vi "solar_cfg String to Variant.vi"(6 "ArrayDelimiters (1D,2D)":string[](array[string]), 8 "error in (no error)":errorcluster, 10 "String":string, 11 "Variant in":variant) -> (0 "error out":errorcluster, 2 "Variant (Binary)":string, 3 "Variant out":variant)   [LabVIEW 2018]
doc: "This converts the ASCII <b>String</b> to <b>Variant out</b> given the <b>Variant in</b> data type."
uses:
  <vilib>/Utility/Data Type/NI_Data Type.lvlib
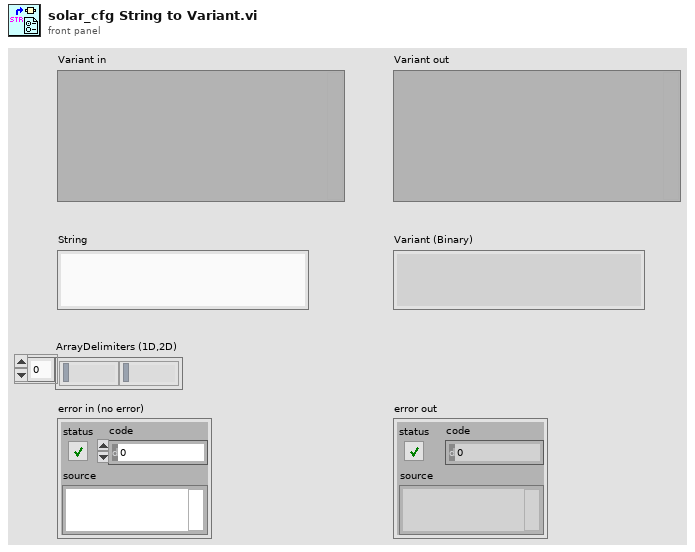
[diagram p1: front panel]
types:
  T1 = typedef "NI_Data Type.lvlib/Data Type.ctl" = enum8{"Invalid Type", "Void", "I8", "I16", "I32", "I64", "U8", "U16", "U32", "U64", "Single Float", "Double Float", "Extended Float", "Single Complex", "Double Complex", "Extended Complex", "Enum U8", "Enum U16", "Enum U32", "Enum U64", "Single Float With Unit", "Double Float With Unit", "Extended Float With Unit", "Single Complex with Unit", "Double Complex with Unit", "Extended Complex with Unit", "Boolean", "String", "Path", "Picture", "Tag", "Array", "Cluster", "Variant", "LV Variant", "Waveform", "Timestamp", "Digital Waveform", "Digital Data", "ExpressData", "Refnum", "External Data", "VI", "Poly VI", "LabVIEW Class Instance", "Fixed Point", "Set Collection", "Map Collection"}
  T2 = typedef "NI_Data Type.lvlib/Refnum Type.ctl" = enum16{"NotARefnum", "UnknownRefnum", "Generic", "Datalog", "ByteStream", "Device", "Occurence", "TCPNetConnection", "Auto", "Menu", "Imaq", "Hardware", "DataSocket", "Visa", "IVI", "UDPNetConnection", "Notifier", "Queue", "Irda", "EventReg", "DotNet", "UserEvent", "Callback", "UNUSED_EMPTY_POSITION", "BlueToothNetConnection", "LVObjApp", "LVObjVI", "LVObjUnknown", "GenericClass", "UserDefinedRefnumTag", "DataValue", "RT FIFO", "TDMS File", "PythonSessionRefnum"}
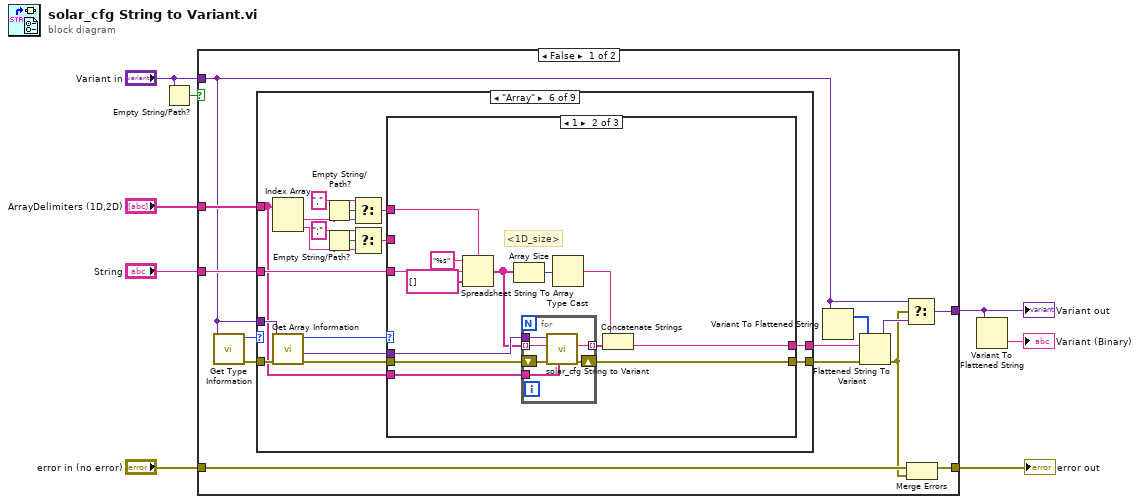
[diagram p0: block diagram]
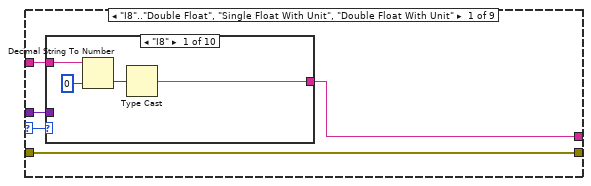
[diagram p2: hidden frame]
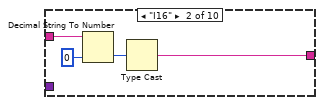
[diagram p3: hidden frame]
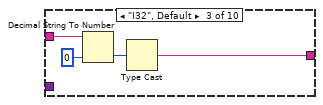
[diagram p4: hidden frame]
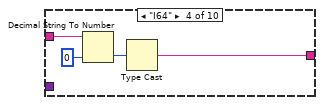
[diagram p5: hidden frame]
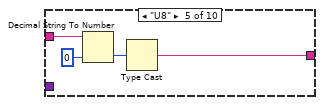
[diagram p6: hidden frame]
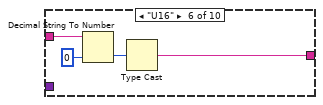
[diagram p7: hidden frame]
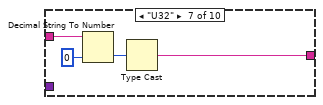
[diagram p8: hidden frame]
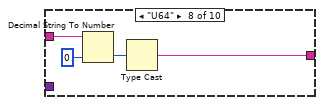
[diagram p9: hidden frame]
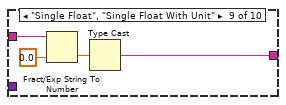
[diagram p10: hidden frame]
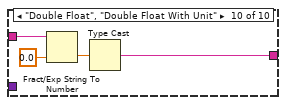
[diagram p11: hidden frame]
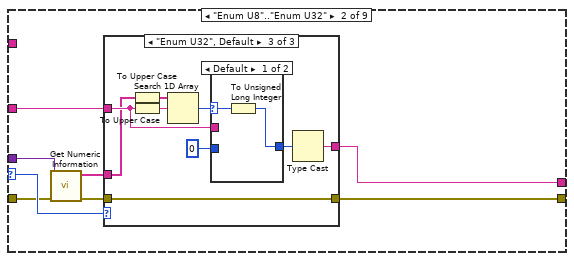
[diagram p12: hidden frame]
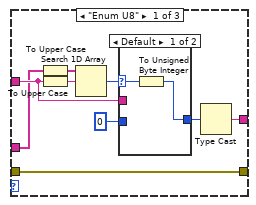
[diagram p13: hidden frame]
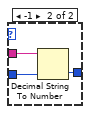
[diagram p14: hidden frame]
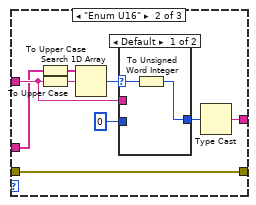
[diagram p15: hidden frame]
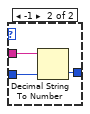
[diagram p16: hidden frame]
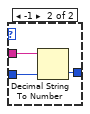
[diagram p17: hidden frame]
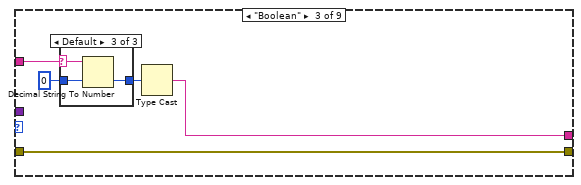
[diagram p18: hidden frame]
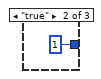
[diagram p20: hidden frame]
diagram:
  n1 = Empty String/Path?(string/path="Variant in") -> (empty?=w1:bool)
  n2 = case shown="False" w1 {
    tunnel: "ArrayDelimiters (1D,2D)" -> [w19 _]
    tunnel: "error in (no error)" -> [w18 w267]
    tunnel: [w17 w267] -> w6
    tunnel: "String" -> [w16 _]
    tunnel: "Variant in" -> [w12 w266]
    tunnel: [w10 w266] -> w3
    frame False {
      n3 = call <vilib>:"Get Type Information.vi"("variant"=w12) -> ("error out"=w20:errorcluster, "type"=w21:T1)  [unwired: 6 in, 3 out]
      n4 = case shown="\"Array\"" w21 {
        selector: w21 -> [w24 w73 _ _ _ _ _ _ _]
        tunnel: w12 -> [w22 w71 _ _ _ w150 _ w229 _]
        tunnel: w20 -> [w26 w72 w118 w128 w135 w153 w223 w230 w258]
        tunnel: [w26 w74 w118 w128 w134 w142 w219 w232 w258] -> w14
        tunnel: [w23 w67 w117 w127 w132 w141 w220 w231 w252] -> w13
        tunnel: w19 -> [_ _ _ _ _ w137 _ _ _]
        tunnel: w16 -> [w25 w68 w119 w129 w133 w139 w222 w226 w253]
        frame "I8".."Double Float", "Single Float With Unit", "Double Float With Unit" {
          n5 = case shown="\"I8\"" w24 {
            tunnel: w25 -> [w28 w32 w36 w40 w44 w48 w52 w56 w61 w65]
            tunnel: [w27 w31 w35 w39 w43 w47 w51 w55 w62 w66] -> w23
            tunnel: w22 -> [_ _ _ _ _ _ _ _ _ _]
            frame "I8" {
              n6 = Decimal String To Number(string=w28, default (0L)=i8 0 ("default (0 I32)")) -> (number=w29:i8)  [unwired: 1 in, 1 out]
              n7 = Type Cast(x=w29) -> (*(type *) &x=w27:string)  [unwired: 1 in]
            }
            frame "I16" {
              n8 = Decimal String To Number(string=w32, default (0L)=i16 0 ("default (0 I32)")) -> (number=w33:i16)  [unwired: 1 in, 1 out]
              n9 = Type Cast(x=w33) -> (*(type *) &x=w31:string)  [unwired: 1 in]
            }
            frame "I32", Default {
              n10 = Decimal String To Number(string=w36, default (0L)=0 ("default (0 I32)")) -> (number=w37:i32)  [unwired: 1 in, 1 out]
              n11 = Type Cast(x=w37) -> (*(type *) &x=w35:string)  [unwired: 1 in]
            }
            frame "I64" {
              n12 = Decimal String To Number(string=w40, default (0L)=i64 0 ("default (0 I32)")) -> (number=w41:i64)  [unwired: 1 in, 1 out]
              n13 = Type Cast(x=w41) -> (*(type *) &x=w39:string)  [unwired: 1 in]
            }
            frame "U8" {
              n14 = Decimal String To Number(string=w44, default (0L)=u8 0 ("default (0 I32)")) -> (number=w45:u8)  [unwired: 1 in, 1 out]
              n15 = Type Cast(x=w45) -> (*(type *) &x=w43:string)  [unwired: 1 in]
            }
            frame "U16" {
              n16 = Decimal String To Number(string=w48, default (0L)=u16 0 ("default (0 I32)")) -> (number=w49:u16)  [unwired: 1 in, 1 out]
              n17 = Type Cast(x=w49) -> (*(type *) &x=w47:string)  [unwired: 1 in]
            }
            frame "U32" {
              n18 = Decimal String To Number(string=w52, default (0L)=u32 0 ("default (0 I32)")) -> (number=w53:u32)  [unwired: 1 in, 1 out]
              n19 = Type Cast(x=w53) -> (*(type *) &x=w51:string)  [unwired: 1 in]
            }
            frame "U64" {
              n20 = Decimal String To Number(string=w56, default (0L)=u64 0 ("default (0 I32)")) -> (number=w57:u64)  [unwired: 1 in, 1 out]
              n21 = Type Cast(x=w57) -> (*(type *) &x=w55:string)  [unwired: 1 in]
            }
            frame "Single Float", "Single Float With Unit" {
              n22 = Fract/Exp String To Number(string=w61, default (0 dbl)=sgl 0.0 ("default (0 I32)")) -> (number=w59:sgl)  [unwired: 2 in, 1 out]
              n23 = Type Cast(x=w59) -> (*(type *) &x=w62:string)  [unwired: 1 in]
            }
            frame "Double Float", "Double Float With Unit" {
              n24 = Fract/Exp String To Number(string=w65, default (0 dbl)=0.0 ("default (0 I32)")) -> (number=w63:dbl)  [unwired: 2 in, 1 out]
              n25 = Type Cast(x=w63) -> (*(type *) &x=w66:string)  [unwired: 1 in]
            }
          }
        }
        frame "Enum U8".."Enum U32" {
          n26 = call <vilib>:"Get Numeric Information.vi"("error in (no error)"=w72, "variant"=w71) -> ("error out"=w70:errorcluster, "enum names"=w69:string[])  [unwired: 6 in, 2 out]
          n27 = case shown="\"Enum U32\", Default" w73 {
            tunnel: w70 -> [w77 w91 w105]
            tunnel: [w77 w91 w105] -> w74
            tunnel: w69 -> [w76 w90 w104]
            tunnel: w68 -> [w78 w92 w106]
            tunnel: [w75 w89 w103] -> w67
            frame "Enum U8" {
              n28 = To Upper Case(1:w76) -> (0:w81:string[])
              n29 = To Upper Case(1:w78) -> (0:w80:string)
              n30 = Search 1D Array(1D array=w81, element=w80) -> (index of element=w82:i32)  [unwired: 1 in]
              n31 = case shown="Default" w82 {
                selector: w82 -> [w85 _]
                tunnel: [w84 w88] -> w83
                tunnel: w78 -> [_ w87]
                tunnel: u8 0 ("default (0 I32)") -> [_ w86]
                frame Default {
                  n32 = To Unsigned Byte Integer(number=w85) -> (unsigned 8bit integer=w84:u8)
                }
                frame -1 {
                  n33 = Decimal String To Number(string=w87, default (0L)=w86) -> (number=w88:u8)  [unwired: 1 in, 1 out]
                }
              }
              n34 = Type Cast(x=w83) -> (*(type *) &x=w75:string)  [unwired: 1 in]
            }
            frame "Enum U16" {
              n35 = To Upper Case(1:w90) -> (0:w95:string[])
              n36 = To Upper Case(1:w92) -> (0:w94:string)
              n37 = Search 1D Array(1D array=w95, element=w94) -> (index of element=w96:i32)  [unwired: 1 in]
              n38 = case shown="Default" w96 {
                selector: w96 -> [w99 _]
                tunnel: [w98 w102] -> w97
                tunnel: w92 -> [_ w101]
                tunnel: u16 0 ("default (0 I32)") -> [_ w100]
                frame Default {
                  n39 = To Unsigned Word Integer(number=w99) -> (unsigned 16bit integer=w98:u16)
                }
                frame -1 {
                  n40 = Decimal String To Number(string=w101, default (0L)=w100) -> (number=w102:u16)  [unwired: 1 in, 1 out]
                }
              }
              n41 = Type Cast(x=w97) -> (*(type *) &x=w89:string)  [unwired: 1 in]
            }
            frame "Enum U32", Default {
              n42 = To Upper Case(1:w104) -> (0:w109:string[])
              n43 = To Upper Case(1:w106) -> (0:w108:string)
              n44 = Search 1D Array(1D array=w109, element=w108) -> (index of element=w110:i32)  [unwired: 1 in]
              n45 = case shown="Default" w110 {
                selector: w110 -> [w113 _]
                tunnel: [w112 w116] -> w111
                tunnel: w106 -> [_ w115]
                tunnel: u32 0 ("default (0 I32)") -> [_ w114]
                frame Default {
                  n46 = To Unsigned Long Integer(number=w113) -> (unsigned 32bit integer=w112:u32)
                }
                frame -1 {
                  n47 = Decimal String To Number(string=w115, default (0L)=w114) -> (number=w116:u32)  [unwired: 1 in, 1 out]
                }
              }
              n48 = Type Cast(x=w111) -> (*(type *) &x=w103:string)  [unwired: 1 in]
            }
          }
        }
        frame "Boolean" {
          n49 = case shown="Default" w119 {
            selector: w119 -> [_ _ w126]
            tunnel: u8 0 ("default (0 I32)") -> [w122 _ w125]
            tunnel: [w122 u8 1 w124] -> w120
            frame "false" {
            }
            frame "true" {
            }
            frame Default {
              n50 = Decimal String To Number(string=w126, default (0L)=w125) -> (number=w124:u8)  [unwired: 1 in, 1 out]
            }
          }
          n51 = Type Cast(x=w120) -> (*(type *) &x=w117:string)  [unwired: 1 in]
        }
        frame "String", "Tag" {
          # "Add length prefix"
          n52 = String Length(string=w129) -> (length=w131:i32)
          n53 = Type Cast(x=w131) -> (*(type *) &x=w130:string)  [unwired: 1 in]
          n54 = Concatenate Strings(w130, w129) -> (w127:string)
        }
        frame "Path" {
          # "PTH0<I32_size>..."
          n55 = String To Path(string=w133) -> (path=w136:path)
          n56 = Flatten To String(anything=w136, error in (no error)=w135) -> (data string=w132:string, error out=w134:errorcluster)  [unwired: 2 in, 1 out]
        }
        frame "Array" {
          n57 = Index Array(array=w137) -> (element #1=w148:string, element #2=w147:string)  [unwired: 2 in]
          n58 = call <vilib>:"Get Array Information.vi"("error in (no error)"=w153, "variant"=w150) -> ("error out"=w151:errorcluster, "array element data type"=w138:variant, "number of dimensions"=w152:i32)  [unwired: 6 in, 1 out]
          n59 = Empty String/Path?(string/path=w148) -> (empty?=w149:bool)
          n60 = Empty String/Path?(string/path=w147) -> (empty?=w145:bool)
          n61 = Select(t=",", s=w149, f=w148) -> (s? t:f=w143:string)
          n62 = Select(t=";", s=w145, f=w147) -> (s? t:f=w140:string)
          n63 = case shown="1" w152 {
            tunnel: w151 -> [w159 w192 w211]
            tunnel: w143 -> [w163 w196 _]
            tunnel: [w158 w191 w211] -> w142
            tunnel: [w160 w193 w205] -> w141
            tunnel: w140 -> [w166 _ _]
            tunnel: w139 -> [w167 w186 w206]
            tunnel: w138 -> [w157 w190 _]
            tunnel: w137 -> [w155 w188 _]
            frame 2 {
              w164 = string[] []
              w165 = "%s" ("format string")
              # "<1D_size><2D_size>..."
              n64 = Spreadsheet String To Array(delimiter (Tab)=w166, format string=w165, spreadsheet string=w167, array type (2D Dbl)=w164) -> (array=w168:string[])
              n65 = for {
                tunnel: w168 -> [w184] mode=indexing
                tunnel: w165 -> [w183]
                tunnel: w164 -> [w185]
                tunnel: w163 -> [w182]
                tunnel: [w181] -> w154 mode=indexing
                n66 = Spreadsheet String To Array(delimiter (Tab)=w182, format string=w183, spreadsheet string=w184, array type (2D Dbl)=w185) -> (array=w181:string[])
              }
              n67 = for {
                shift-right: [w173] -> w158
                shift-left: w159 -> [w174]
                tunnel: w157 -> [w172]
                tunnel: w154 -> [w171] mode=indexing
                tunnel: [w170] -> w156 mode=concatenating
                tunnel: w155 -> [w169]
                n68 = for {
                  tunnel: w172 -> [w178]
                  tunnel: w171 -> [w177] mode=indexing
                  tunnel: [w176] -> w170 mode=indexing
                  tunnel: w169 -> [w175]
                  shift-right: [w179] -> w173
                  shift-left: w174 -> [w180]
                  n69 = call "solar_cfg String to Variant.vi"("ArrayDelimiters (1D,2D)"=w175, "error in (no error)"=w180, "String"=w177, "Variant in"=w178) -> ("error out"=w179:errorcluster, "Variant (Binary)"=w176:string)  [unwired: 5 in, 1 out]
                }
              }
              n70 = Array Size(array=w154) -> (size(s)=w161:i32[])
              n71 = Type Cast(x=w161) -> (*(type *) &x=w162:string)  [unwired: 1 in]
              n72 = Concatenate Strings(w162, w156) -> (w160:string)
            }
            frame 1 {
              # "<1D_size>"
              n73 = Spreadsheet String To Array(delimiter (Tab)=w196, format string="%s", spreadsheet string=w186, array type (2D Dbl)=string[] []) -> (array=w187:string[])
              n74 = Array Size(array=w187) -> (size(s)=w194:i32)
              n75 = for {
                shift-right: [w203] -> w191
                shift-left: w192 -> [w204]
                tunnel: w190 -> [w202]
                tunnel: w187 -> [w201] mode=indexing
                tunnel: [w200] -> w189 mode=indexing
                tunnel: w188 -> [w199]
                n76 = call "solar_cfg String to Variant.vi"("ArrayDelimiters (1D,2D)"=w199, "error in (no error)"=w204, "String"=w201, "Variant in"=w202) -> ("error out"=w203:errorcluster, "Variant (Binary)"=w200:string)  [unwired: 5 in, 1 out]
              }
              n77 = Type Cast(x=w194) -> (*(type *) &x=w195:string)  [unwired: 1 in]
              n78 = Concatenate Strings(w195, w189) -> (w193:string)
            }
            frame Default {
              w210 = 2 ("y")
              n79 = String Length(string=w206) -> (length=w208:i32)
              n80 = Quotient & Remainder(x=w208, y=w210) -> (floor(x/y)=w209:i32)  [unwired: 1 out]
              n81 = for {
                N: w209 -> [_]
                tunnel: w206 -> [w218]
                tunnel: [w213] -> w207 mode=indexing
                tunnel: w210 -> [w212]
                i -> [w217]
                n82 = Multiply(x=w217, y=w212) -> (x*y=w216:i32)
                n83 = String Subset(string=w218, offset (0)=w216, length (rest)=w212) -> (substring=w215:string)
                n84 = Hexadecimal String To Number(string=w215, default (0uL)=u8 0 ("default (0 U32)")) -> (number=w213:u8)  [unwired: 1 in, 1 out]
              }
              n85 = Byte Array To String(unsigned byte array=w207) -> (string=w205:string)
            }
          }
        }
        frame "Timestamp" {
          # "16 bytes"
          n86 = Scan From String(format string="%<%Y-%m-%d_%H:%M:%S%6u>T", input string=w222, error in=w223, default 1=timestamp(0 s since 1904-01-01)) -> (error out=w219:errorcluster, output 1=w224:timestamp)  [unwired: 1 in, 2 out]
          n87 = Flatten To String(anything=w224) -> (data string=w220:string)  [unwired: 3 in, 2 out]
        }
        frame "Refnum" {
          n88 = call <vilib>:"Get Refnum Information.vi"("error in (no error)"=w230, "variant"=w229) -> ("error out"=w228:errorcluster, "reference type"=w227:T2)  [unwired: 6 in, 2 out]
          n89 = case shown="\"Visa\"" w227 {
            tunnel: [w239 w248] -> w232
            tunnel: [w233 w247] -> w231
            tunnel: w229 -> [_ _]
            tunnel: w228 -> [w239 w248]
            tunnel: w226 -> [w234 w249]
            frame Default {
              w238 = 2 ("y")
              n90 = String Length(string=w234) -> (length=w236:i32)
              n91 = Quotient & Remainder(x=w236, y=w238) -> (floor(x/y)=w237:i32)  [unwired: 1 out]
              n92 = for {
                N: w237 -> [_]
                tunnel: w234 -> [w246]
                tunnel: [w241] -> w235 mode=indexing
                tunnel: w238 -> [w240]
                i -> [w245]
                n93 = Multiply(x=w245, y=w240) -> (x*y=w244:i32)
                n94 = String Subset(string=w246, offset (0)=w244, length (rest)=w240) -> (substring=w243:string)
                n95 = Hexadecimal String To Number(string=w243, default (0uL)=u8 0 ("default (0 U32)")) -> (number=w241:u8)  [unwired: 1 in, 1 out]
              }
              n96 = Byte Array To String(unsigned byte array=w235) -> (string=w233:string)
            }
            frame "Visa" {
              # "Add length prefix"
              n97 = String Length(string=w249) -> (length=w251:i32)
              n98 = Type Cast(x=w251) -> (*(type *) &x=w250:string)  [unwired: 1 in]
              n99 = Concatenate Strings(w250, w249) -> (w247:string)
            }
          }
        }
        frame Default {
          w257 = 2 ("y")
          n100 = String Length(string=w253) -> (length=w255:i32)
          n101 = Quotient & Remainder(x=w255, y=w257) -> (floor(x/y)=w256:i32)  [unwired: 1 out]
          n102 = for {
            N: w256 -> [_]
            tunnel: w253 -> [w265]
            tunnel: [w260] -> w254 mode=indexing
            tunnel: w257 -> [w259]
            i -> [w264]
            n103 = Multiply(x=w264, y=w259) -> (x*y=w263:i32)
            n104 = String Subset(string=w265, offset (0)=w263, length (rest)=w259) -> (substring=w262:string)
            n105 = Hexadecimal String To Number(string=w262, default (0uL)=u8 0 ("default (0 U32)")) -> (number=w260:u8)  [unwired: 1 in, 1 out]
          }
          n106 = Byte Array To String(unsigned byte array=w254) -> (string=w252:string)
        }
      }
      n107 = Variant To Flattened String(Variant=w12) -> (1:w15:i16[])  [unwired: 1 out]
      n108 = Flattened String To Variant(4:w14, 6:w13, 7:w15) -> (0:w9:errorcluster, 3:w11:variant)
      n109 = Select(t=w12, s=w9, f=w11) -> (s? t:f=w10:variant)
      n110 = Merge Errors(w18, w9) -> (w17:errorcluster)
    }
    frame True {
    }
  }
  "error out" <- w6
  "Variant out" <- w3
  n111 = Variant To Flattened String(Variant=w3) -> (data string=→"Variant (Binary)":string)  [unwired: 1 out]
